vi "VI Anlagengrenzwerte PNS.vi"() -> ()   [LabVIEW 2020, in "PNS.lvlib"]
uses:
  PNS/PNS.lvlib
  PNS/Anlagengrenzwerte PNS.ctl
  PNS/Anlagengrenzwerte-Parameter Anzeige.ctl
  Visualisierungs Elemente/Zahlen-Eingabefeld.ctl
  Visualisierungs Elemente/Button.ctl
  Visualisierungs Elemente/Zahlen-Ausgabefeld.ctl
  PNS/PNS Istwerte.ctl
  PNS/Aktionen FGV Grenzwerte.ctl
  PNS/Aktionen FGV Loopkennung.ctl
  PNS/PNS Anlagenuebersicht einfaerben Aktionen.ctl
  Passwortverwaltung/FGV Passwort Aktion.ctl
  PNS/Komm Modbus/Aktionen FGV Komm MB.ctl
  PNS/Aktionen FGV Istwerte.ctl
  PNS/Aktion FGV AO PNS.ctl
  PNS/Diagnose PNS.vi
  Passwortverwaltung/Passwort.lvlib
  Allgemein/allgemeine Sub-VIs.lvlib
  PNS/Komm Modbus/Modbus TypDef.lvlib
  PNS/Komm Modbus/Komm Modbus.lvlib
panel:
  out "AO PROP":u16
  out "max Lops":T1 caption="max Lops:" format="%#_5g"
  in  "IP-Adresse PNS:":string
  out "Software Version:":string
  out "PNS Istwerte":T2 {"Istwert 8" format="%.1f"; "Istwert 7" format="%.1f"; "Istwert 6" format="%.1f"; "Istwert 5" format="%.1f"; "Istwert 4" format="%.1f"; "Istwert 3" format="%.1f"; "Istwert 2" format="%.1f"; "Istwert 1" format="%.1f"}
  out "Seriennummer:":string
  out "Gerätetyp:":string
  out "Detail Status:":T1 format="%#_5g"
  out "Status:":T1 format="%#_5g"
  out "Druckluft Störung:":T1 format="%#_5g"
  out "AWC IST:":T1 format="%#_5g"
  out "AWC Soll:":T1 format="%#_5g"
  out "Error Out":errorcluster caption="Fehlercluster"
  in  "Diag PNS":T3
  in  "Grenzwerte PNS":T4={"Filter:"={"Sollwert"=0.0, "Warn-Min"=0.0, "Warn-Max"=0.0, "Abschalt-Min"=0.0, "Abschalt-Max"=0.0, "Regler"=1, "AnlagenParameter"=""}, "Ventilplatte:"={"Sollwert"=0.0, "Warn-Min"=0.0, "Warn-Max"=0.0, "Abschalt-Min"=0.0, "Abschalt-Max"=0.0, "Regler"=1, "AnlagenParameter"=""}, "Heizleitung 1:"={"Sollwert"=0.0, "Warn-Min"=0.0, "Warn-Max"=0.0, "Abschalt-Min"=0.0, "Abschalt-Max"=0.0, "Regler"=1, "AnlagenParameter"=""}, "Heizleitung 2:"={"Sollwert"=0.0, "Warn-Min"=0.0, "Warn-Max"=0.0, "Abschalt-Min"=0.0, "Abschalt-Max"=0.0, "Regler"=1, "AnlagenParameter"=""}, "Heizleitung 3:"={"Sollwert"=0.0, "Warn-Min"=0.0, "Warn-Max"=0.0, "Abschalt-Min"=0.0, "Abschalt-Max"=0.0, "Regler"=1, "AnlagenParameter"=""}, "Heizleitung 4:"={"Sollwert"=0.0, "Warn-Min"=0.0, "Warn-Max"=0.0, "Abschalt-Min"=0.0, "Abschalt-Max"=0.0, "Regler"=1, "AnlagenParameter"=""}, "Heizleitung 5:"={"Sollwert"=0.0, "Warn-Min"=0.0, "Warn-Max"=0.0, "Abschalt-Min"=0.0, "Abschalt-Max"=0.0, "Regler"=1, "AnlagenParameter"=""}, "Heizleitung 6:"={"Sollwert"=0.0, "Warn-Min"=0.0, "Warn-Max"=0.0, "Abschalt-Min"=0.0, "Abschalt-Max"=0.0, "Regler"=1, "AnlagenParameter"=""}} {"Heizleitung 6:"."Regler" items=["aktiv", "inaktiv"]; "Heizleitung 6:"."Abschalt-Max" format="%#_5g"; "Heizleitung 6:"."Abschalt-Min" format="%#_5g"; "Heizleitung 6:"."Warn-Max" format="%#_5g"; "Heizleitung 6:"."Warn-Min" format="%#_5g"; "Heizleitung 6:"."Sollwert" format="%#_5g"; "Heizleitung 5:"."Regler" items=["aktiv", "inaktiv"]; "Heizleitung 5:"."Abschalt-Max" format="%#_5g"; "Heizleitung 5:"."Abschalt-Min" format="%#_5g"; "Heizleitung 5:"."Warn-Max" format="%#_5g"; "Heizleitung 5:"."Warn-Min" format="%#_5g"; "Heizleitung 5:"."Sollwert" format="%#_5g"; "Heizleitung 4:"."Regler" items=["aktiv", "inaktiv"]; "Heizleitung 4:"."Abschalt-Max" format="%#_5g"; "Heizleitung 4:"."Abschalt-Min" format="%#_5g"; "Heizleitung 4:"."Warn-Max" format="%#_5g"; "Heizleitung 4:"."Warn-Min" format="%#_5g"; "Heizleitung 4:"."Sollwert" format="%#_5g"; "Heizleitung 3:"."Regler" items=["aktiv", "inaktiv"]; "Heizleitung 3:"."Abschalt-Max" format="%#_5g"; "Heizleitung 3:"."Abschalt-Min" format="%#_5g"; "Heizleitung 3:"."Warn-Max" format="%#_5g"; "Heizleitung 3:"."Warn-Min" format="%#_5g"; "Heizleitung 3:"."Sollwert" format="%#_5g"; "Heizleitung 2:"."Regler" items=["aktiv", "inaktiv"]; "Heizleitung 2:"."Abschalt-Max" format="%#_5g"; "Heizleitung 2:"."Abschalt-Min" format="%#_5g"; "Heizleitung 2:"."Warn-Max" format="%#_5g"; "Heizleitung 2:"."Warn-Min" format="%#_5g"; "Heizleitung 2:"."Sollwert" format="%#_5g"; "Heizleitung 1:"."Regler" items=["aktiv", "inaktiv"]; "Heizleitung 1:"."Abschalt-Max" format="%#_5g"; "Heizleitung 1:"."Abschalt-Min" format="%#_5g"; "Heizleitung 1:"."Warn-Max" format="%#_5g"; "Heizleitung 1:"."Warn-Min" format="%#_5g"; "Heizleitung 1:"."Sollwert" format="%#_5g"; "Ventilplatte:"."Regler" items=["aktiv", "inaktiv"]; "Ventilplatte:"."Abschalt-Max" format="%#_5g"; "Ventilplatte:"."Abschalt-Min" format="%#_5g"; "Ventilplatte:"."Warn-Max" format="%#_5g"; "Ventilplatte:"."Warn-Min" format="%#_5g"; "Ventilplatte:"."Sollwert" format="%#_5g"; "Filter:"."Regler" items=["aktiv", "inaktiv"]; "Filter:"."Abschalt-Max" format="%#_5g"; "Filter:"."Abschalt-Min" format="%#_5g"; "Filter:"."Warn-Max" format="%#_5g"; "Filter:"."Warn-Min" format="%#_5g"; "Filter:"."Sollwert" format="%#_5g"}
  # "Anlagengrenzwerte PNS"
  # "Abschaltgrenzen"
  # "Warngrenzen"
  # "Regelung \naktiv/inaktiv"
  # "Parameter"
  # "Istwert"
  # "Sollwert"
  # "Min"
  # "Max"
  # "Min"
  # "Max"
  # "Allgemeine Werte"
  # "Status Kommunikation"
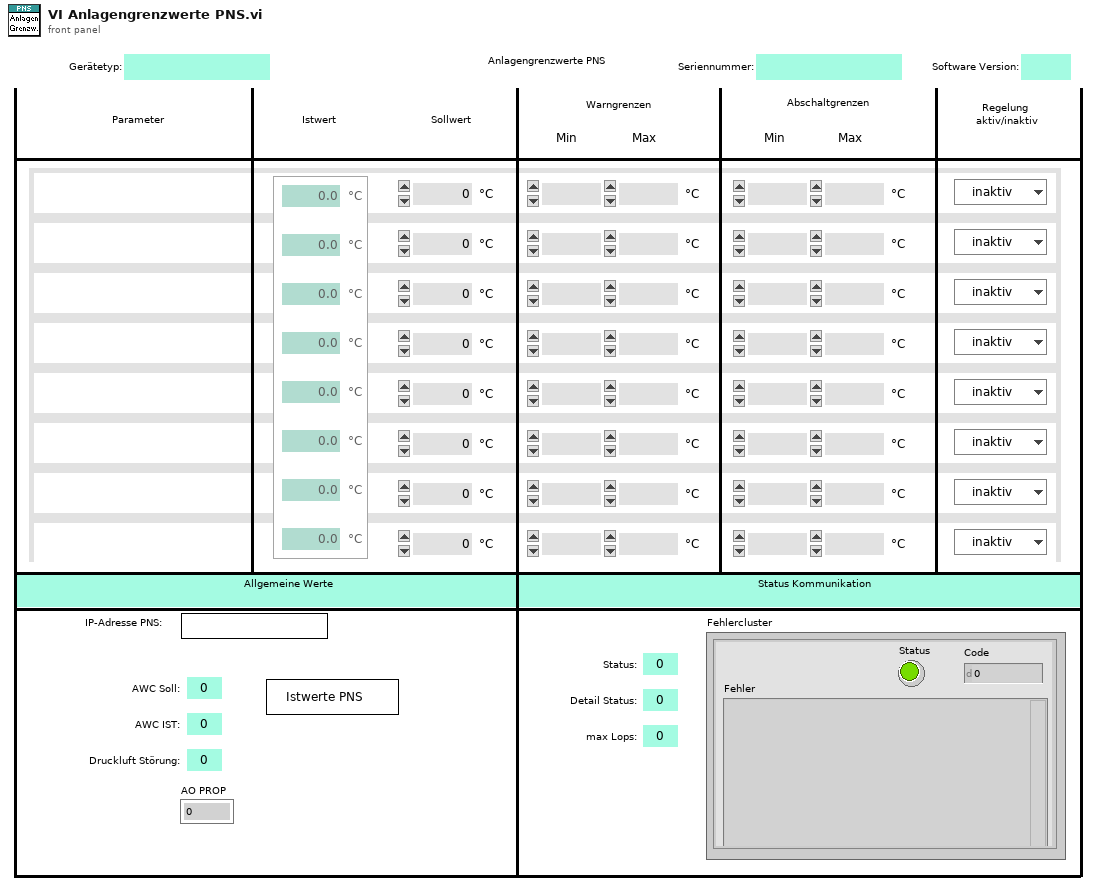
[diagram p1: front panel]
types:
  T1 = typedef "Zahlen-Ausgabefeld.ctl" = sgl
  T2 = typedef "PNS.lvlib/PNS Istwerte.ctl" = cluster{"Istwert 1":sgl, "Istwert 2":sgl, "Istwert 3":sgl, "Istwert 4":sgl, "Istwert 5":sgl, "Istwert 6":sgl, "Istwert 7":sgl, "Istwert 8":sgl}
  T3 = typedef "Button.ctl" = bool
  T4 = typedef "PNS.lvlib/Anlagengrenzwerte PNS.ctl" = cluster{"Filter:":T5, "Ventilplatte:":T5, "Heizleitung 1:":T5, "Heizleitung 2:":T5, "Heizleitung 3:":T5, "Heizleitung 4:":T5, "Heizleitung 5:":T5, "Heizleitung 6:":T5}
  T5 = typedef "PNS.lvlib/Anlagengrenzwerte-Parameter Anzeige.ctl" = cluster{"Sollwert":T6, "Warn-Min":T6, "Warn-Max":T6, "Abschalt-Min":T6, "Abschalt-Max":T6, "Regler":u16, "AnlagenParameter":string}
  T6 = typedef "Zahlen-Eingabefeld.ctl" = sgl
  T7 = typedef "PNS.lvlib/PNS Anlagenuebersicht einfaerben Aktionen.ctl" = enum16{"lesen", "prüfen", "initialisieren"}
  T8 = typedef "PNS.lvlib/Aktionen FGV Loopkennung.ctl" = enum16{"lesen", "schreiben"}
  T9 = typedef "PNS.lvlib/Aktionen FGV Grenzwerte.ctl" = enum16{"lesen", "Grenzw. schreiben", "Anweisungscode", "IP-Adresse", "laden", "speichern", "Anweisungscode vorgeben"}
  T10 = typedef "Steuerung PNS.lvclass/Anlegengrenzwerte PNS.ctl" = cluster{"Filter:":T11, "Ventilplatte:":T11, "Heizleitung 1:":T11, "Heizleitung 2:":T11, "Heizleitung 3:":T11, "Heizleitung 4:":T11, "Heizleitung 5:":T11, "Heizleitung 6:":T11}
  T11 = typedef "Steuerung PNS.lvclass/Anlagengrenzwerte Parameteranzeige.ctl" = cluster{"Sollwert":T6, "Warn-Min":T6, "Warn-Max":T6, "Abschalt-Min":T6, "Abschalt-Max":T6, "Regler":u16, "AnlagenParameter":string}
  T12 = typedef "PNS.lvlib/PNS Geraetekennung.ctl" = cluster{"Loops":string[], "Gerätetype":string, "Loopkennung":u16[], "Seriennummer":string, "Geraetekennung":u16, "SoftWare Version":string, "LP Kennung":u16}
  T13 = typedef "Passwort.lvlib/FGV Passwort Aktion.ctl" = enum16{"prüfen", "setzen", "Initialisieren", "PW speichern", "lesen", "PW Änderung"}
  T14 = typedef "PNS.lvlib/Aktion FGV AO PNS.ctl" = enum16{"lesen", "schreiben"}
  T15 = typedef "PNS.lvlib/Aktionen FGV Istwerte.ctl" = enum16{"lesen", "initialisieren", "schreiben", "Störungen"}
  T16 = typedef "PNS.lvlib/Komm Modbus.lvlib/Modbus TypDef.lvlib/Aktionen FGV Komm MB.ctl" = enum16{"initialisieren", "lesen", "Verbindung herstellen", "Verbindung beenden", "Komm Modbus", "Sollwerte vorgeben", "change lang"}
  T17 = typedef "Steuerung PNS.lvclass/Regler.ctl" = cluster{"Istwert":i16, "Sollwert":i16, "Alarm MIN":i16, "Alarm MAX":i16, "Regler sperren":i16, "Analog Ausgang":i16}[]
  T18 = cluster{"Istwert":i16, "Sollwert":i16, "Alarm MIN":i16, "Alarm MAX":i16, "Regler sperren":i16, "Analog Ausgang":i16}
  T19 = cluster{"Istwert":i16, "Istwert":i16, "Istwert":i16, "Istwert":i16, "Istwert":i16, "Istwert":i16, "Istwert":i16, "Istwert":i16}
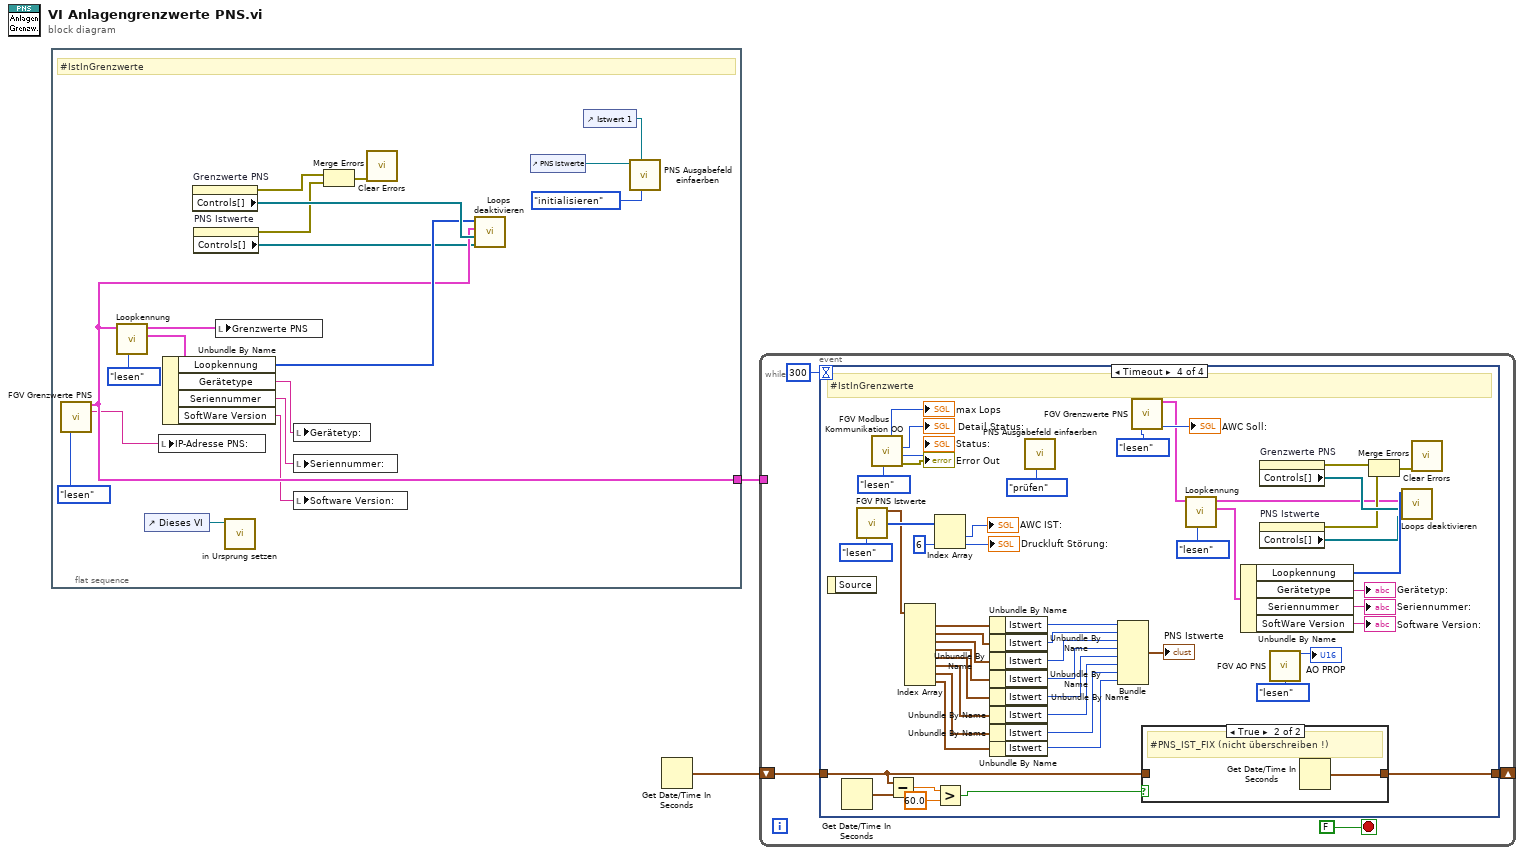
[diagram p0: block diagram]
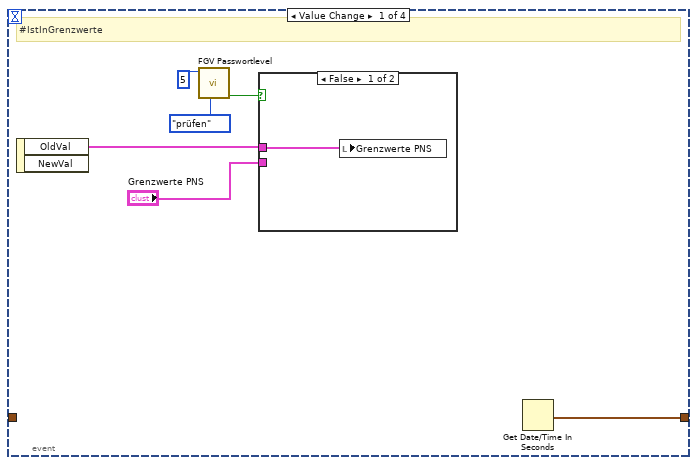
[diagram p2: hidden frame]
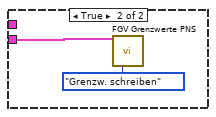
[diagram p3: hidden frame]
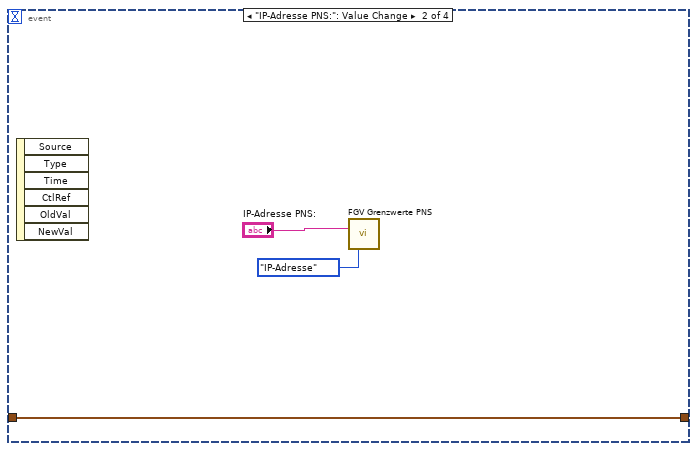
[diagram p4: hidden frame]
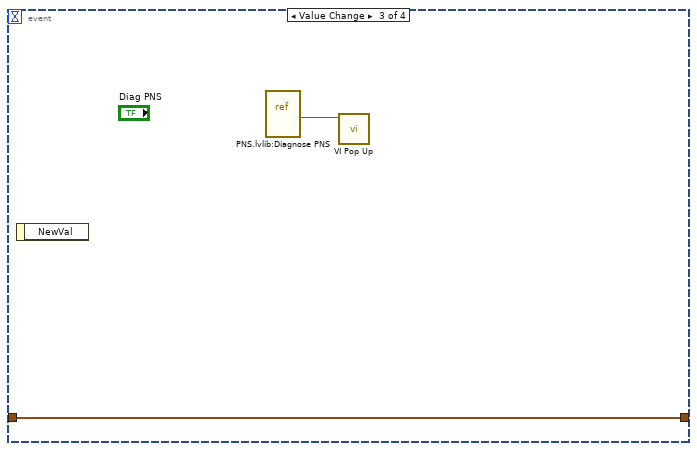
[diagram p5: hidden frame]
diagram:
  n1 = flat-sequence {
    tunnel: [w12] -> w2
    frame #0 {
      # "#IstInGrenzwerte"
      n2 = call "FGV Grenzwerte PNS.vi"("Aktionen FGV Grenzwerte"=Aktionen_FGV_Grenzwerte."lesen") -> ("Grenzwerte PNS 2"=w12:T10, "IP-Adresse"=w3:string)  [unwired: 12 in, 1 out]
      n3 = call "Loopkennung.vi"("Aktion"=Aktionen_FGV_Loopkennung."lesen", "Grenzwerte PNS 2"=w12) -> ("LoopGeraetekennung"=w17:T12, "Grenzwerte PNS"=w19:T10)  [unwired: 8 in]
      n4 = control-ref of="Dieses VI"() -> (w20:refnum<vi>)
      n5 = local write "IP-Adresse PNS:"(w3) -> ()
      n6 = Unbundle By Name(w17) -> ("Loopkennung"=w13:u16[], "Gerätetype"=w16:string, "Seriennummer"=w15:string, "SoftWare Version"=w10:string)
      n7 = property on="Grenzwerte PNS" class="Cluster (strikt)"() -> (error out=w7:errorcluster, "Controls[]"=w14:refnum<vi>[])  [unwired: 2 in, 1 out]
      n8 = property on="PNS Istwerte" class="Cluster (strikt)"() -> (error out=w8:errorcluster, "Controls[]"=w9:refnum<vi>[])  [unwired: 2 in, 1 out]
      n9 = local write "Grenzwerte PNS"(w19) -> ()
      n10 = call "in Ursprung setzen.vi"("VI Referenz"=w20) -> ()  [unwired: 10 in, 1 out]
      n11 = local write "Gerätetyp:"(w16) -> ()
      n12 = local write "Seriennummer:"(w15) -> ()
      n13 = local write "Software Version:"(w10) -> ()
      n14 = Merge Errors(w7, w8) -> (w11:errorcluster)
      n15 = call <vilib>:"Clear Errors.vi"("error in (no error)"=w11) -> ()  [unwired: 5 in, 2 out]
      n16 = call "Loops deaktivieren.vi"("Istwert Controls[]"=w9, "Grenzwert Controls[]"=w14, "Grenzwerte PNS"=w12, "Loopkennung"=w13) -> ()  [unwired: 8 in]
      n17 = control-ref of="PNS Istwerte"() -> (w5:refnum<vi>)
      n18 = control-ref of="Istwert 1"() -> (w4:refnum<vi>)
      n19 = call "PNS Ausgabefeld einfaerben.vi"("Aktionen"=PNS_Anlagenuebersicht_einfaerben_Aktionen."initialisieren", "FeldTyp (Eingang)"=w4, "PNS Istwerte"=w5) -> ()  [unwired: 9 in]
    }
  }
  n20 = Get Date/Time In Seconds() -> (seconds since 1Jan1904=w1:timestamp)
  n21 = while {
    tunnel: w2 -> [_]
    shift-right: [w22] -> _
    shift-left: w1 -> [w23]
    stop <- FALSE stop-if-true
    n22 = event shown="[3] Timeout" {
      selector: _ -> [_ _ _ _]
      dyn-events: _ -> [_ _ _ _]
      timeout: 300 -> [_ _ _ _]
      tunnel: w23 -> [_ w36 w38 w58]
      tunnel: [w26 w36 w38 w57] -> w22
      event Value Change {
        # "#IstInGrenzwerte"
        n23 = event-data() -> ("OldVal"=w28:T4)  [unwired: 2 out]
        n24 = call "FGV Passwortlevel.vi"("FGV Passwort Aktion"=FGV_Passwort_Aktion."prüfen", "geforderter Level"=i16 5) -> ("Freigabe"=w29:bool)  [unwired: 2 in, 7 out]
        n25 = case shown="False" w29 {
          tunnel: "Grenzwerte PNS" -> [_ w33]
          tunnel: w28 -> [w32 _]
          frame False {
            n26 = local write "Grenzwerte PNS"(w32) -> ()
          }
          frame True {
            n27 = call "FGV Grenzwerte PNS.vi"("Grenzwerte PNS"=w33, "Aktionen FGV Grenzwerte"=Aktionen_FGV_Grenzwerte."Grenzw. schreiben") -> ()  [unwired: 11 in, 3 out]
          }
        }
        n28 = Get Date/Time In Seconds() -> (seconds since 1Jan1904=w26:timestamp)
      }
      event "IP-Adresse PNS:": Value Change {
        n29 = event-data() -> ()  [unwired: 7 out]
        n30 = call "FGV Grenzwerte PNS.vi"("IP-Adresse"="IP-Adresse PNS:", "Aktionen FGV Grenzwerte"=Aktionen_FGV_Grenzwerte."IP-Adresse") -> ()  [unwired: 11 in, 3 out]
      }
      event Value Change {
        n31 = event-data() -> ()  [unwired: 2 out]
        n32 = vi-ref "PNS.lvlib:Diagnose PNS.vi"() -> (w39:refnum<vi>)
        n33 = call "VI Pop Up.vi"("VI Referenz"=w39) -> ()  [unwired: 10 in, 1 out]
      }
      event Timeout {
        # "#IstInGrenzwerte"
        n34 = event-data() -> ()  [unwired: 2 out]
        n35 = Get Date/Time In Seconds() -> (seconds since 1Jan1904=w62:timestamp)
        n36 = call "FGV PNS Istwerte.vi"("Aktionen"=Aktionen_FGV_Istwerte."lesen") -> ("Regler"=w63:T17, "UsrVal"=w81:u16[])  [unwired: 11 in, 2 out]
        n37 = call "FGV Modbus Kommunikation OO.vi"("Aktionen"=Aktionen_FGV_Komm_MB."lesen") -> ("Fehler (Ausgang)"=→"Error Out":errorcluster, "Index"=→"Status:":u8, "Case Nr."=→"Detail Status:":u8, "maxLoop"=→"max Lops":u8)  [unwired: 4 in, 1 out]
        n38 = Subtract(x=w58, y=w62) -> (x-y=w61:dbl)
        n39 = Index Array(array=w63) -> (element #1=w80:T18, element #2=w79:T18, element #3=w78:T18, element #4=w76:T18, element #5=w77:T18, element #6=w75:T18, element #7=w74:T18, element #8=w66:T18)  [unwired: 8 in]
        n40 = Index Array(array=w81, index #2=6 ("Index")) -> (element #1=→"AWC IST:":u16, element #2=→"Druckluft Störung:":u16)  [unwired: 1 in]
        n41 = Greater?(x=w61, y=60.0) -> (0:w59:bool)
        n42 = Unbundle By Name(w80) -> ("Istwert"=w73:i16)
        n43 = Unbundle By Name(w79) -> ("Istwert"=w72:i16)
        n44 = Unbundle By Name(w78) -> ("Istwert"=w71:i16)
        n45 = Unbundle By Name(w76) -> ("Istwert"=w70:i16)
        n46 = Unbundle By Name(w77) -> ("Istwert"=w69:i16)
        n47 = Unbundle By Name(w75) -> ("Istwert"=w68:i16)
        n48 = Unbundle By Name(w74) -> ("Istwert"=w67:i16)
        n49 = Unbundle By Name(w66) -> ("Istwert"=w65:i16)
        n50 = call "PNS Ausgabefeld einfaerben.vi"("Aktionen"=PNS_Anlagenuebersicht_einfaerben_Aktionen."prüfen") -> ()  [unwired: 11 in]
        n51 = Bundle("Istwert"=w73, "Istwert"=w72, "Istwert"=w71, "Istwert"=w70, "Istwert"=w69, "Istwert"=w68, "Istwert"=w67, "Istwert"=w65) -> (→"PNS Istwerte":T19)  [unwired: 1 in]
        n52 = call "FGV Grenzwerte PNS.vi"("Aktionen FGV Grenzwerte"=Aktionen_FGV_Grenzwerte."lesen") -> ("Grenzwerte PNS 2"=w42:T10, "Anweisungscode"=→"AWC Soll:":u16)  [unwired: 12 in, 1 out]
        n53 = case shown="True" w59 {
          tunnel: w58 -> [w92 _]
          tunnel: [w92 w93] -> w57
          frame False {
          }
          frame True {
            # "#PNS_IST_FIX (nicht überschreiben !)"
            n54 = Get Date/Time In Seconds() -> (seconds since 1Jan1904=w93:timestamp)
          }
        }
        n55 = call "Loopkennung.vi"("Aktion"=Aktionen_FGV_Loopkennung."lesen", "Grenzwerte PNS 2"=w42) -> ("LoopGeraetekennung"=w55:T12, "Grenzwerte PNS"=w45:T10)  [unwired: 8 in]
        n56 = Unbundle By Name(w55) -> ("Loopkennung"=w51:u16[], "Gerätetype"=→"Gerätetyp:":string, "Seriennummer"=→"Seriennummer:":string, "SoftWare Version"=→"Software Version:":string)
        n57 = property on="Grenzwerte PNS" class="Cluster (strikt)"() -> (error out=w47:errorcluster, "Controls[]"=w49:refnum<vi>[])  [unwired: 2 in, 1 out]
        n58 = property on="PNS Istwerte" class="Cluster (strikt)"() -> (error out=w46:errorcluster, "Controls[]"=w50:refnum<vi>[])  [unwired: 2 in, 1 out]
        n59 = call "FGV AO PNS.vi"("Aktion"=Aktion_FGV_AO_PNS."lesen") -> ("AO PROP"=→"AO PROP":u16)  [unwired: 13 in, 1 out]
        n60 = Merge Errors(w47, w46) -> (w48:errorcluster)
        n61 = call "Loops deaktivieren.vi"("Istwert Controls[]"=w50, "Grenzwert Controls[]"=w49, "Grenzwerte PNS"=w45, "Loopkennung"=w51) -> ()  [unwired: 8 in]
        n62 = call <vilib>:"Clear Errors.vi"("error in (no error)"=w48) -> ()  [unwired: 5 in, 2 out]
      }
    }
  }
